vi "Parse Metric.vi"(10 "Metric name":string, 11 "String":string) -> (3 "Metric properties":T1)   [LabVIEW 2015, in "NI_Azure_Blob.lvlib"]
uses:
  NI_Azure_Blob.lvlib
  Metrics.ctl
  Retention Policy.ctl
  XML Parsing/NI_Azure_XML Parsing.lvlib
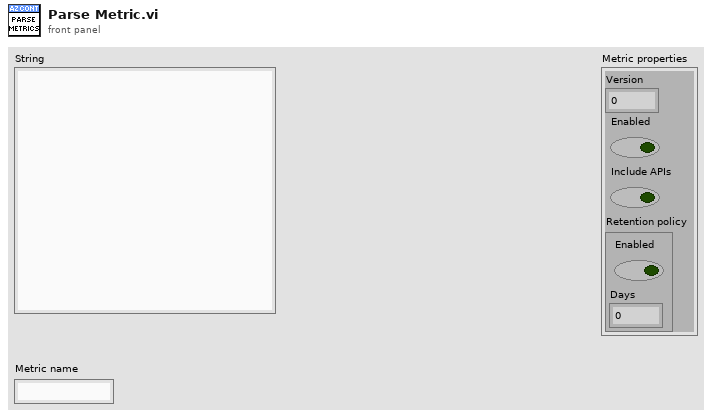
[diagram p1: front panel]
types:
  T1 = typedef "NI_Azure_Blob.lvlib/Metrics.ctl" = cluster{"Version":dbl, "Enabled":bool, "Include APIs":bool, "Retention policy":T2}
  T2 = typedef "NI_Azure_Blob.lvlib/Retention Policy.ctl" = cluster{"Enabled":bool, "Days":u32}
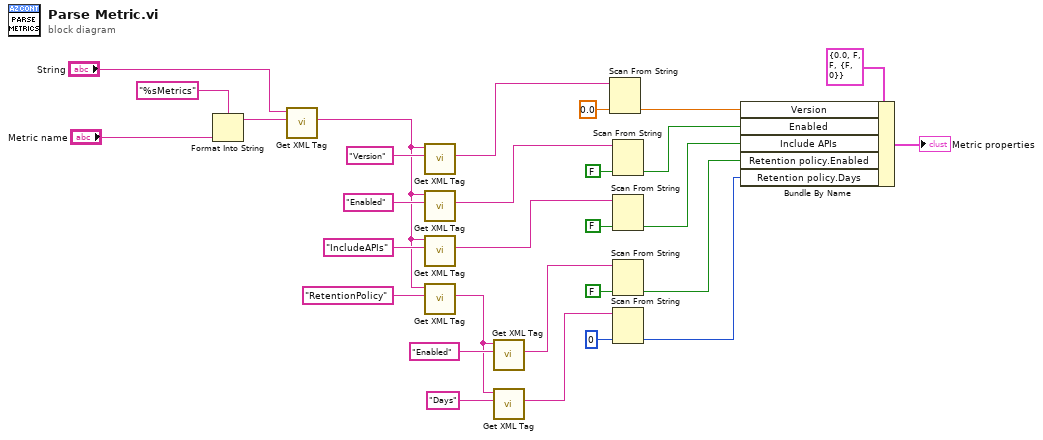
[diagram p0: block diagram]
diagram:
  n1 = Format Into String(format string="%sMetrics", "Metric name") -> (resulting string=w29:string)  [unwired: 2 in, 1 out]
  n2 = call "Get XML Tag.vi"("Tag name"=w29, "XML String in"="String") -> ("Tag value"=w18:string)  [unwired: 5 in, 4 out]
  n3 = call "Get XML Tag.vi"("Tag name"="Version", "XML String in"=w18) -> ("Tag value"=w8:string)  [unwired: 5 in, 4 out]
  n4 = call "Get XML Tag.vi"("Tag name"="Enabled", "XML String in"=w18) -> ("Tag value"=w10:string)  [unwired: 5 in, 4 out]
  n5 = call "Get XML Tag.vi"("Tag name"="IncludeAPIs", "XML String in"=w18) -> ("Tag value"=w11:string)  [unwired: 5 in, 4 out]
  n6 = call "Get XML Tag.vi"("Tag name"="RetentionPolicy", "XML String in"=w18) -> ("Tag value"=w19:string)  [unwired: 5 in, 4 out]
  n7 = call "Get XML Tag.vi"("Tag name"="Enabled", "XML String in"=w19) -> ("Tag value"=w14:string)  [unwired: 5 in, 4 out]
  n8 = call "Get XML Tag.vi"("Tag name"="Days", "XML String in"=w19) -> ("Tag value"=w15:string)  [unwired: 5 in, 4 out]
  n9 = Scan From String(input string=w8, default 1=0.0 ("Version")) -> (output 1=w6:dbl)  [unwired: 3 in, 3 out]
  n10 = Scan From String(input string=w10, default 1=FALSE) -> (output 1=w5:bool)  [unwired: 3 in, 3 out]
  n11 = Scan From String(input string=w11, default 1=FALSE) -> (output 1=w4:bool)  [unwired: 3 in, 3 out]
  n12 = Scan From String(input string=w14, default 1=FALSE) -> (output 1=w3:bool)  [unwired: 3 in, 3 out]
  n13 = Scan From String(input string=w15, default 1=u32 0 ("Retention policy.Days")) -> (output 1=w2:u32)  [unwired: 3 in, 3 out]
  n14 = Bundle By Name(cluster=T1 {"Version"=0.0, "Enabled"=FALSE, "Include APIs"=FALSE, "Retention policy"={"Enabled"=FALSE, "Days"=0}} ("Metric properties"), "Version"=w6, "Enabled"=w5, "Include APIs"=w4, "Retention policy.Enabled"=w3, "Retention policy.Days"=w2) -> (→"Metric properties":T1)
